vi "Main.vi"() -> ()   [LabVIEW 2015, in "SR430Class.lvclass"]
doc: "This template is for the Queued Message Handler design pattern.\n\nThe Event Handling Loop generates messages based on user interface actions.\n\nThe Message Handling Loop processes messages generated by the Event Handling Loop, or by other messages. The messages are string values, so new messages can be added easily to the Message Cases case structure in the Message Handling Loop. Each message cluster can also provide an optional value for Message Data, which is a variant that can be converted to whatever message-specific data is required."
uses:
  class/SR430Class.lvclass
  support/Type Definitions/Export.ctl
  support/Type Definitions/Mode.ctl
  support/Type Definitions/Schedule.ctl
  support/Type Definitions/saveGraph.ctl
  class/SR430Class.lvclass/SR430Class.ctl
  support/SR430 Driver/SR430_VISA Control.ctl
  support/Message Queue/Enqueue Message (Single).vi
  <vilib>/Utility/error.llb/Error Cluster From Error Code.vi
  <vilib>/ErrorRing/Error Ring.xnode
  support/Message Queue/Message Queue.lvlib
  support/User Event - Stop/User Event - Stop.lvlib
  support/SR430 Driver/SR430Driver.lvlib
  support/Error Handling/Error Handling.lvlib
  support/Type Definitions/Type Definition.lvlib
panel:
  in  "Save":T1
  in  "Schedule":T2 caption="Open"
  in  "Mode":T3 caption="Config"
  in  "Excel Export":T4 caption="New"
  in  "VISA resource name":refnum<visa-resource-name>="Select COM Port"
  in  "Blink":bool caption="Blank"
  in  "Abort":bool
  in  "Accept Mode":bool caption="Blank"
  out "Display":string caption="String"
  in  "Start Timed Acq.":bool caption="Blank"
  in  "TRIGGER LEVEL":dbl=0.1 caption="Numeric" min=-2.0 max=2.0
  in  "DISCRIM. LEVEL":dbl=-0.3 caption="Numeric" min=-0.3 max=0.3
  in  "BINS/RECORD":i32=1 caption="Numeric" min=1 max=16
  in  "RECORDS/SCAN":i32=1000 caption="Numeric" min=0 max=655355
  in  "BIN WIDTH":i32 caption="Numeric" min=0 max=19
  in  "TRIGGER OFFSET":i32=1 caption="Numeric" min=0 max=16384 step=16
  in  "Clock":bool caption="Blank"
  in  "Discrim Slope":bool caption="Blank"
  in  "Trigger Slope":bool=TRUE caption="Blank"
  in  "Startup Banner 2":string="Architect: Ryan J. Richards\nSupervising Professor: Dr. TIm Kane\nThe Pennsylvania State University" caption="String"
  out "ID":string caption="String"
  in  "Startup Banner":string="Stanford Research Systems\nModel SR430 Multi-Channel Scaler | Photon Counter" caption="String"
  in  "Seconds":dbl caption="Numeric" min=0.0
  in  "Minutes":dbl caption="Numeric" min=0.0
  in  "Acquitision Iteration":i32=1 caption="Numeric" min=1
  in  "Hours":dbl caption="Numeric" min=0.0
  out "SR430 Output":dbl[][](graph)
  in  "Clear":bool caption="Reset"
  in  "Pause":bool
  in  "Start":bool
  in  "SR430 Resource":refnum<class "SR430Class.lvclass">
  # "TIMED ACQUISITION"
  # "SYSTEM SETTINGS"
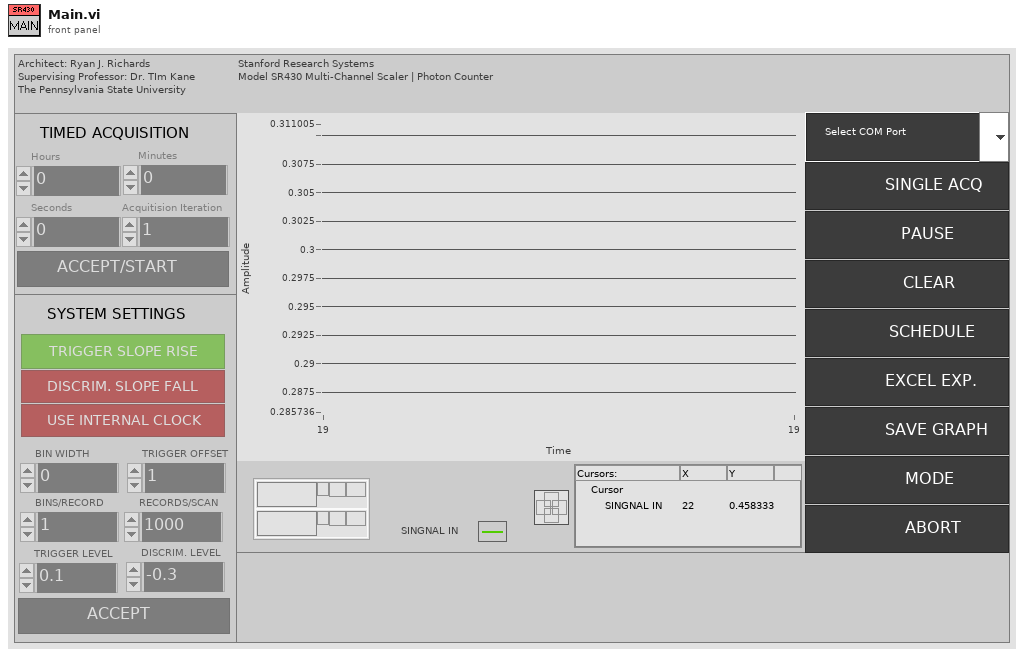
[diagram p1: front panel]
types:
  T1 = typedef "Type Definition.lvlib/saveGraph.ctl" = bool
  T2 = typedef "Type Definition.lvlib/Schedule.ctl" = bool
  T3 = typedef "Type Definition.lvlib/Mode.ctl" = bool
  T4 = typedef "Type Definition.lvlib/Export.ctl" = bool
  T5 = typedef "Message Queue.lvlib/All Message Queues.ctl" = cluster{"UI":refnum<queue>}
  T6 = enum8{"Enabled", "Disabled", "Disabled and Grayed Out"}
  T7 = typedef "SR430Driver.lvlib/SR430_VISA Control.ctl" = cluster{"VISA resource name":refnum<visa-resource-name>}
  T8 = cluster{"Trigger Level (V)":dbl, "Discriminator Level (V)":dbl, "Trigger Slope":bool, "Disc. Slope":bool, "Use External Clock":bool, "Bin Width":i32, "Bins/Record":i32, "Records/Scan":i32, "Trigger Offset":i32}
  T9 = cluster{"Hours":dbl, "Minutes":dbl, "Seconds":dbl, "ACQ #:":i32}
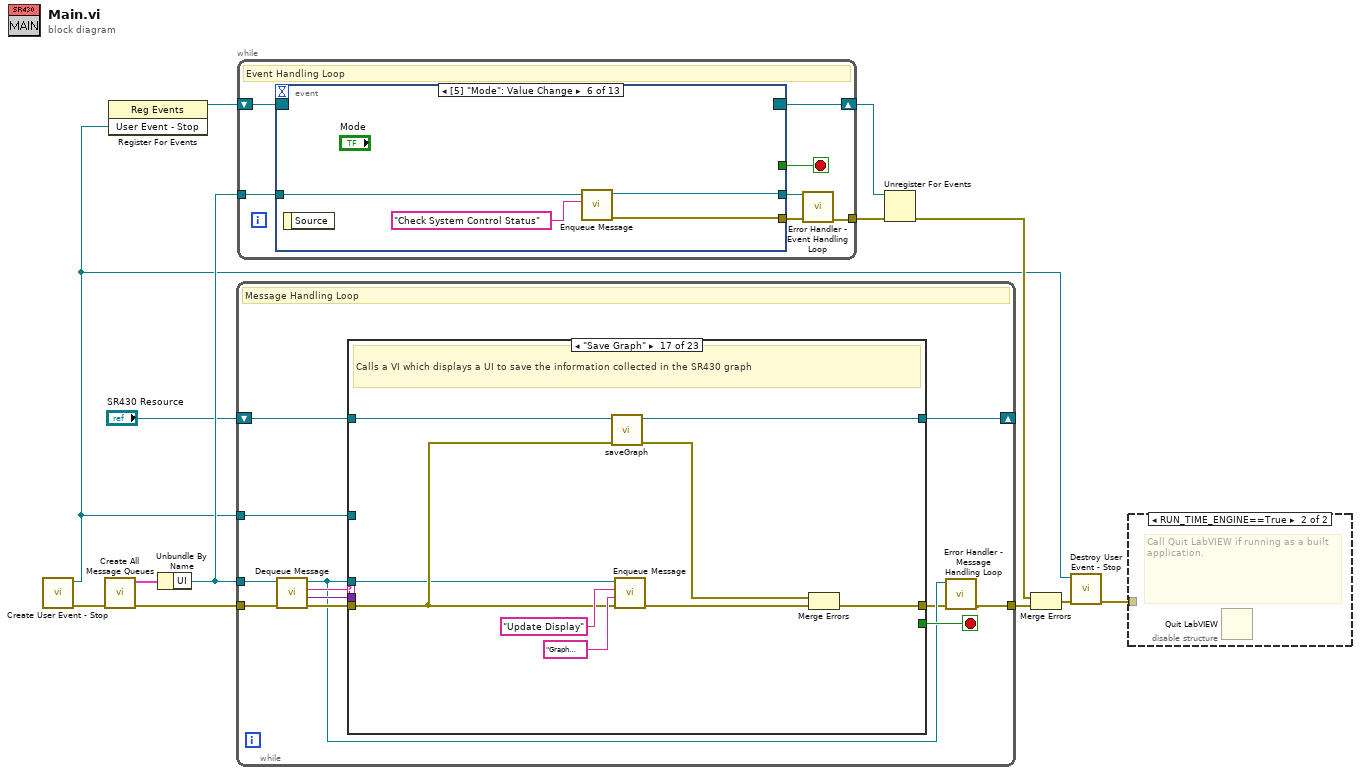
[diagram p0: block diagram]
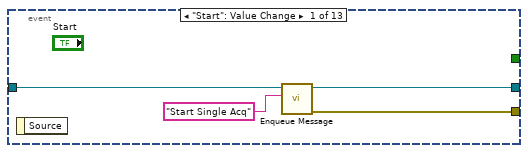
[diagram p3: hidden frame]
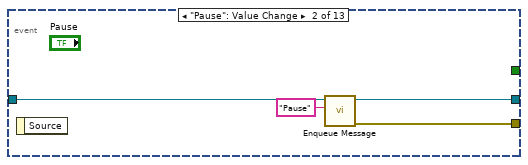
[diagram p4: hidden frame]
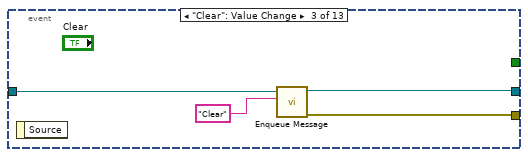
[diagram p5: hidden frame]
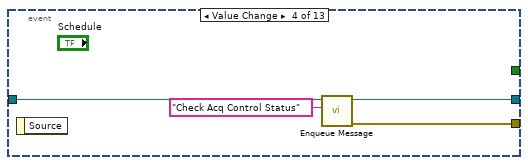
[diagram p6: hidden frame]
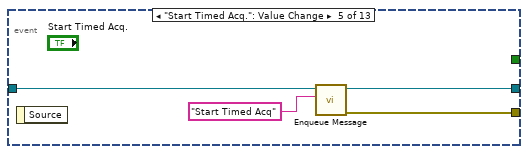
[diagram p7: hidden frame]
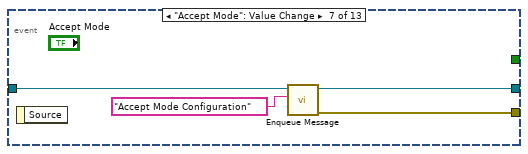
[diagram p8: hidden frame]
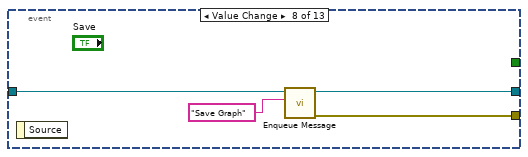
[diagram p9: hidden frame]
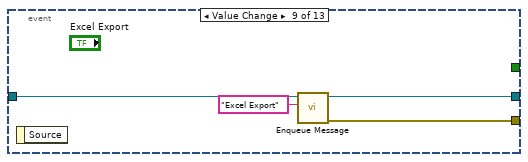
[diagram p10: hidden frame]
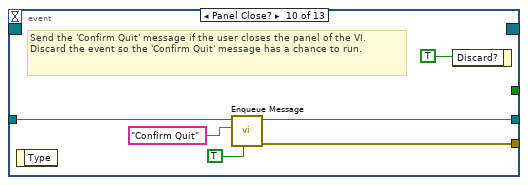
[diagram p11: hidden frame]
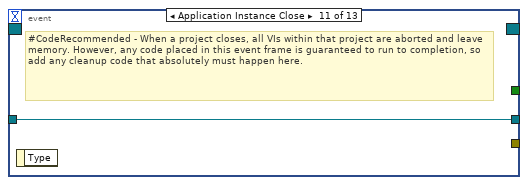
[diagram p12: hidden frame]
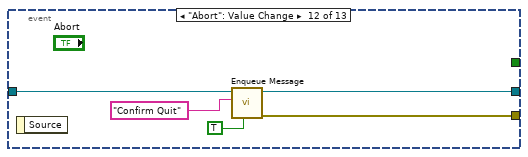
[diagram p13: hidden frame]
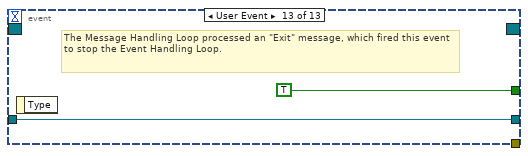
[diagram p14: hidden frame]
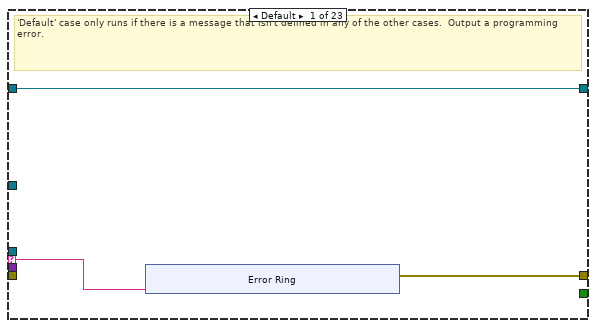
[diagram p15: hidden frame]
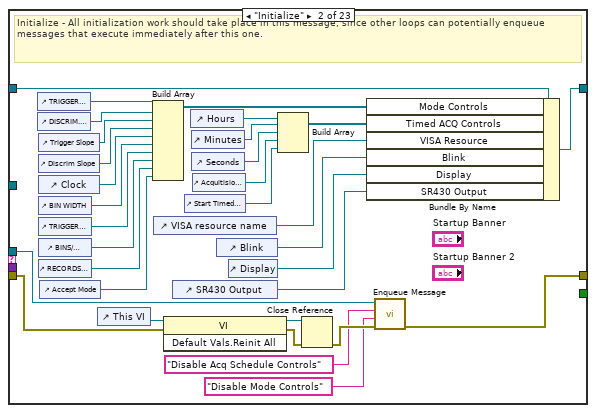
[diagram p16: hidden frame]
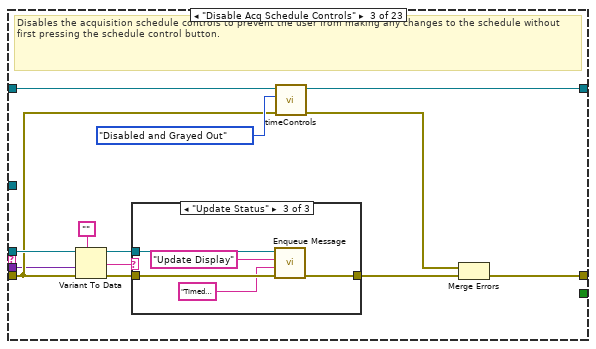
[diagram p17: hidden frame]
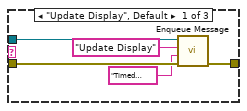
[diagram p18: hidden frame]
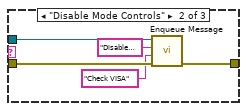
[diagram p19: hidden frame]
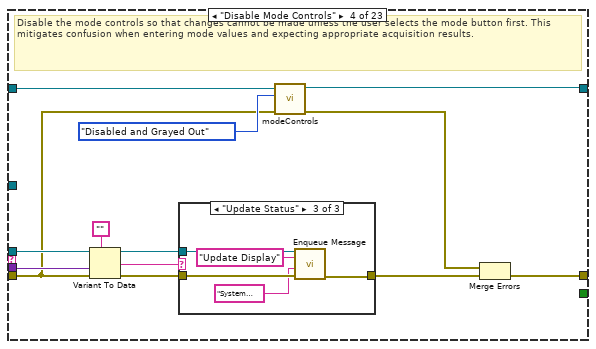
[diagram p20: hidden frame]
diagram:
  n1 = call "Create User Event - Stop.vi"() -> ("error out"=w9:errorcluster, "User Event - Stop"=w3:refnum<user-event>)  [unwired: 10 in]
  n2 = call "Create All Message Queues.vi"("error in (no error)"=w9) -> ("error out"=w13:errorcluster, "Message Queues out"=w12:T5)  [unwired: 9 in]
  n3 = register-events(w3) -> (reference out=w4:refnum<event-registration>)  [unwired: 2 in, 1 out]
  n4 = Unbundle By Name(w12) -> ("UI"=w10:refnum<queue>)
  n5 = while {
    tunnel: w10 -> [w17]
    shift-right: [w24] -> _
    shift-left: "SR430 Resource" -> [w25]
    tunnel: w3 -> [w22]
    tunnel: w13 -> [w21]
    tunnel: [w14] -> w11
    stop <- w23 stop-if-true
    # "Message Handling Loop"
    n6 = call "Dequeue Message.vi"("error in (no error)"=w21, "Message Queue"=w17) -> ("error out"=w20:errorcluster, "Message Data"=w18:variant, "Message"=w19:string, "dup Message Queue"=w16:refnum<queue>)  [unwired: 6 in]
    n7 = case "Message Cases" shown="\"Save Graph\"" w19 {
      selector: w19 -> [w26 _ _ _ _ _ _ _ _ _ _ _ _ _ _ _ _ _ _ _ _ _ _]
      tunnel: w16 -> [_ w59 w70 w103 w126 w144 w155 w170 w178 w188 w215 w226 w234 _ w252 w259 w263 w277 _ w293 _ w306 w328]
      tunnel: w20 -> [_ w64 w69 w96 w125 w143 w150 w166 w177 w187 w216 w222 w235 w245 w251 w260 w266 w278 w285 w292 w303 w305 w321]
      tunnel: [w27 w60 w75 w100 w121 w136 w152 w167 w174 w183 w212 w228 w230 w244 w248 w256 w264 w272 w286 w290 w298 w304 w324] -> w15
      tunnel: w25 -> [w28 w67 w79 w106 w128 w146 w158 w173 w182 w194 w219 w224 w242 w247 w255 w262 w271 w280 w287 w295 w302 w311 w327]
      tunnel: [w28 w66 w78 w105 w127 w145 w157 w172 w181 w193 w218 w223 w241 w246 w254 w262 w270 w279 w287 w294 w302 w311 w327] -> w24
      tunnel: [_ _ _ _ _ _ _ _ _ _ _ _ _ _ _ _ _ _ _ _ _ _ TRUE] -> w23
      tunnel: w18 -> [_ _ w68 w98 _ _ w148 _ _ w186 _ _ _ _ _ _ _ _ w284 _ w301 _ w318]
      tunnel: w22 -> [_ _ _ _ _ _ _ _ _ _ _ _ _ _ _ _ _ _ _ _ _ _ w323]
      frame Default {
        # "'Default' case only runs if there is a message that isn't defined in any of the other cases.  Output a programming error."
        n8 = xnode "Error Ring"("parameter 0"=w26) -> ("error out"=w27:errorcluster)
      }
      frame "Initialize" {
        # "Initialize - All initialization work should take place in this message, since other loops can potentially enqueue messages that execute immediately after this one."
        n9 = control-ref of="TRIGGER LEVEL"() -> (w55:refnum<vi>)
        n10 = control-ref of="DISCRIM. LEVEL"() -> (w54:refnum<vi>)
        n11 = control-ref of="Trigger Slope"() -> (w53:refnum<vi>)
        n12 = control-ref of="Discrim Slope"() -> (w52:refnum<vi>)
        n13 = control-ref of="Clock"() -> (w51:refnum<vi>)
        n14 = control-ref of="BIN WIDTH"() -> (w50:refnum<vi>)
        n15 = control-ref of="TRIGGER OFFSET"() -> (w49:refnum<vi>)
        n16 = control-ref of="BINS/RECORD"() -> (w48:refnum<vi>)
        n17 = control-ref of="RECORDS/SCAN"() -> (w47:refnum<vi>)
        n18 = control-ref of="Accept Mode"() -> (w45:refnum<vi>)
        n19 = control-ref of="This VI"() -> (w65:refnum<vi>)
        n20 = Build Array(w55, w54, w53, w52, w51, w50, w49, w48, w47, w45) -> (w46:refnum<vi>[])
        n21 = control-ref of="VISA resource name"() -> (w57:refnum<vi>)
        n22 = invoke class="VI" method="Default Vals.Reinit All"(reference=w65, error in=w64) -> (reference out=w63:refnum<vi>, error out=w62:errorcluster)  [unwired: 1 in, 1 out]
        n23 = control-ref of="SR430 Output"() -> (w36:refnum<vi>)
        n24 = control-ref of="Start Timed Acq."() -> (w39:refnum<vi>)
        n25 = control-ref of="Hours"() -> (w44:refnum<vi>)
        n26 = control-ref of="Minutes"() -> (w43:refnum<vi>)
        n27 = control-ref of="Seconds"() -> (w42:refnum<vi>)
        n28 = control-ref of="Acquitision Iteration"() -> (w41:refnum<vi>)
        n29 = control-ref of="Blink"() -> (w56:refnum<vi>)
        n30 = control-ref of="Display"() -> (w38:refnum<vi>)
        n31 = Build Array(w44, w43, w42, w41, w39) -> (w40:refnum<vi>[])
        n32 = Close Reference(reference=w63, error in (no error)=w62) -> (error out=w61:errorcluster)
        n33 = Bundle By Name(cluster=w67, "Mode Controls"=w46, "Timed ACQ Controls"=w40, "VISA Resource"=w57, "Blink"=w56, "Display"=w38, "SR430 Output"=w36) -> (w66:refnum<class "SR430Class.lvclass">)
        n34 = call-poly "Enqueue Message.vi"("error in (no error)"=w61, "Message Data"="Disable Mode Controls" ("Message"), "Message"="Disable Acq Schedule Controls", "Message Queue"=w59) -> ("error out"=w60:errorcluster)  [unwired: 6 in, 1 out]
      }
      frame "Disable Acq Schedule Controls" {
        # "Disables the acquisition schedule controls to prevent the user from making any changes to the schedule without first pressing the schedule control button."
        n35 = Variant To Data(error in=w69, type="", Variant=w68) -> (data=w73:string, error out=w72:errorcluster)
        n36 = case shown="\"Update Status\"" w73 {
          tunnel: w72 -> [w83 w89 w94]
          tunnel: w70 -> [w84 w88 w92]
          tunnel: [w81 w86 w93] -> w71
          frame "Update Display", Default {
            n37 = call-poly "Enqueue Message.vi"("error in (no error)"=w83, "Message Data"="Timed acquisition process complete" ("Message"), "Message"="Update Display", "Message Queue"=w84) -> ("error out"=w81:errorcluster)  [unwired: 6 in, 1 out]
          }
          frame "Disable Mode Controls" {
            n38 = call-poly "Enqueue Message.vi"("error in (no error)"=w89, "Message Data"="Check VISA" ("Message"), "Message"="Disable Mode Controls", "Message Queue"=w88) -> ("error out"=w86:errorcluster)  [unwired: 6 in, 1 out]
          }
          frame "Update Status" {
            n39 = call-poly "Enqueue Message.vi"("error in (no error)"=w94, "Message Data"="Timed ACQ Controls Disabled" ("Message"), "Message"="Update Display", "Message Queue"=w92) -> ("error out"=w93:errorcluster)  [unwired: 6 in, 1 out]
          }
        }
        n40 = call-dynamic "timeControls.vi"("error in (no error)"=w69, "Enabled/Disabled"=T6."Disabled and Grayed Out", "SR430Class in"=w79) -> ("error out"=w76:errorcluster, "SR430Class out"=w78:refnum<class "SR430Class.lvclass">)  [unwired: 7 in]
        n41 = Merge Errors(w76, w71) -> (w75:errorcluster)
      }
      frame "Disable Mode Controls" {
        # "Disable the mode controls so that changes cannot be made unless the user selects the mode button first. This mitigates confusion when entering mode values and expecting appropriate acquisition results."
        n42 = Variant To Data(error in=w96, type="", Variant=w98) -> (data=w97:string, error out=w95:errorcluster)
        n43 = case shown="\"Update Status\"" w97 {
          tunnel: w95 -> [w110 w115 w119]
          tunnel: w103 -> [w111 w114 w120]
          tunnel: [w107 w112 w118] -> w102
          frame "Update Display", Default {
            n44 = call-poly "Enqueue Message.vi"("error in (no error)"=w110, "Message Data"="System settings have been updated." ("Message"), "Message"="Update Display", "Message Queue"=w111) -> ("error out"=w107:errorcluster)  [unwired: 6 in, 1 out]
          }
          frame "Check VISA" {
            n45 = call-poly "Enqueue Message.vi"("error in (no error)"=w115, "Message"="Check VISA", "Message Queue"=w114) -> ("error out"=w112:errorcluster)  [unwired: 7 in, 1 out]
          }
          frame "Update Status" {
            n46 = call-poly "Enqueue Message.vi"("error in (no error)"=w119, "Message Data"="System settings controls disabled." ("Message"), "Message"="Update Display", "Message Queue"=w120) -> ("error out"=w118:errorcluster)  [unwired: 6 in, 1 out]
          }
        }
        n47 = call "modeControls.vi"("error in (no error)"=w96, "Enabled/Disabled"=T6."Disabled and Grayed Out", "SR430Class in"=w106) -> ("error out"=w101:errorcluster, "SR430Class out"=w105:refnum<class "SR430Class.lvclass">)  [unwired: 7 in]
        n48 = Merge Errors(w101, w102) -> (w100:errorcluster)
      }
      frame "Check VISA" {
        # "Checks the VISA control to determine whether or not a COM port has been selected (other than default value). If it has not then the control will blink and require the user to change the port and select a valid one"
        n49 = call-dynamic "checkVisa.vi"("error in (no error)"=w125, "SR430Class in"=w128) -> ("error out"=w123:errorcluster, "SR430Class out"=w127:refnum<class "SR430Class.lvclass">)  [unwired: 8 in]
        n50 = call-poly "Enqueue Message.vi"("error in (no error)"=w125, "Message"="Initialize SR430", "Message Queue"=w126) -> ("error out"=w122:errorcluster)  [unwired: 7 in, 1 out]
        n51 = Merge Errors(w123, w122) -> (w121:errorcluster)
      }
      frame "Initialize SR430" {
        # "Provide the VISA resource so that the SR430 can connect to LabVIEW. The connection status and identification number is then displayed accordingly."
        n52 = Bundle By Name(cluster=T7 {"VISA resource name"=""} ("SR430 VISA Cluster"), "VISA resource name"="VISA resource name") -> (w129:T7)
        n53 = call-dynamic "initializeSR430.vi"("error in (no error)"=w143, "SR430 VISA Cluster"=w129, "dataClass in"=w146) -> ("error out"=w135:errorcluster, "ID #:"=w133:string, "Connected"=w141:bool, "dataClass out"=w145:refnum<class "SR430Class.lvclass">)  [unwired: 5 in]
        n54 = Select(t="Connected to SR430" ("Message"), s=w141, f="Failed to connect to SR430" ("Message")) -> (s? t:f=w139:string)
        n55 = Concatenate Strings("Connected to:" ("string"), w133) -> (→"ID":string)
        n56 = call-poly "Enqueue Message.vi"("error in (no error)"=w143, "Message Data"=w139, "Message"="Update Display", "Message Queue"=w144) -> ("error out"=w137:errorcluster)  [unwired: 6 in, 1 out]
        n57 = Merge Errors(w135, w137) -> (w136:errorcluster)
      }
      frame "Enable Mode Controls" {
        # "Enable Mode Controls so that the user can change them and ultimately accept the configuration. This prevents the user from changing them during execution and mitigates confusion and error."
        n58 = Variant To Data(error in=w150, type="", Variant=w148) -> (data=w147:string, error out=w149:errorcluster)
        n59 = case shown="\"Update Status\"" w147 {
          tunnel: w149 -> [w159 w164]
          tunnel: w155 -> [_ w163]
          tunnel: [w159 w160] -> w154
          frame Default {
          }
          frame "Update Status" {
            n60 = call-poly "Enqueue Message.vi"("error in (no error)"=w164, "Message Data"="System settings controls enabled." ("Message"), "Message"="Update Display", "Message Queue"=w163) -> ("error out"=w160:errorcluster)  [unwired: 6 in, 1 out]
          }
        }
        n61 = call "modeControls.vi"("error in (no error)"=w150, "Enabled/Disabled"=T6."Enabled", "SR430Class in"=w158) -> ("error out"=w153:errorcluster, "SR430Class out"=w157:refnum<class "SR430Class.lvclass">)  [unwired: 7 in]
        n62 = Merge Errors(w153, w154) -> (w152:errorcluster)
      }
      frame "Check Acq Control Status" {
        # "Checks the status of the acquisition controls and reads whether they are enabled or disabled - then assigns the next state accordingly."
        n63 = call-dynamic "CheckControlStatus.vi"("error in (no error)"=w166, "SR430Class in"=w173) -> ("error out"=w168:errorcluster, "Enable/Disable Controls"=w171:string, "SR430Class out"=w172:refnum<class "SR430Class.lvclass">)  [unwired: 7 in]
        n64 = call-poly "Enqueue Message.vi"("error in (no error)"=w166, "Message Data"="Update Status" ("Enable/Disable Controls"), "Message"=w171, "Message Queue"=w170) -> ("error out"=w169:errorcluster)  [unwired: 6 in, 1 out]
        n65 = Merge Errors(w168, w169) -> (w167:errorcluster)
      }
      frame "Check System Control Status" {
        # "Checks the status of the system settings controls and reads whether they are enabled or disabled - then assigns the next state accordingly."
        n66 = call-dynamic "CheckSystemSettingControl.vi"("error in (no error)"=w177, "SR430Class in"=w182) -> ("error out"=w176:errorcluster, "Enable/Disable Controls"=w179:string, "SR430Class out"=w181:refnum<class "SR430Class.lvclass">)  [unwired: 7 in]
        n67 = call-poly "Enqueue Message.vi"("error in (no error)"=w177, "Message Data"="Update Status" ("Enable/Disable Controls"), "Message"=w179, "Message Queue"=w178) -> ("error out"=w175:errorcluster)  [unwired: 6 in, 1 out]
        n68 = Merge Errors(w176, w175) -> (w174:errorcluster)
      }
      frame "Enable Acq Schedule Controls" {
        # "Enables the acqusition schedule controls so that the user can enter the desired time values and execute the acquisition process."
        n69 = Variant To Data(error in=w187, type="", Variant=w186) -> (data=w190:string, error out=w189:errorcluster)
        n70 = case shown="\"Update Status\"" w190 {
          tunnel: w189 -> [w195 w200]
          tunnel: w188 -> [_ w198]
          tunnel: [w195 w199] -> w185
          frame Default {
          }
          frame "Update Status" {
            n71 = call-poly "Enqueue Message.vi"("error in (no error)"=w200, "Message Data"="Timed ACQ Controls Enabled." ("Message"), "Message"="Update Display", "Message Queue"=w198) -> ("error out"=w199:errorcluster)  [unwired: 6 in, 1 out]
          }
        }
        n72 = call-dynamic "timeControls.vi"("error in (no error)"=w187, "Enabled/Disabled"=T6."Enabled", "SR430Class in"=w194) -> ("error out"=w184:errorcluster, "SR430Class out"=w193:refnum<class "SR430Class.lvclass">)  [unwired: 7 in]
        n73 = Merge Errors(w184, w185) -> (w183:errorcluster)
      }
      frame "Accept Mode Configuration" {
        # "Writes the mode values to the SR430, effectively updating the settings on the device so that a specific acquisition can be completed."
        n74 = Bundle By Name(cluster=T8 {"Trigger Level (V)"=0.1, "Discriminator Level (V)"=-0.3, "Trigger Slope"=FALSE, "Disc. Slope"=TRUE, "Use External Clock"=FALSE, "Bin Width"=0, "Bins/Record"=1, "Records/Scan"=1000, "Trigger Offset"=0}, "Trigger Level (V)"="TRIGGER LEVEL", "Discriminator Level (V)"="DISCRIM. LEVEL", "Trigger Slope"="Trigger Slope", "Disc. Slope"="Discrim Slope", "Use External Clock"="Clock", "Bin Width"="BIN WIDTH", "Bins/Record"="BINS/RECORD", "Records/Scan"="RECORDS/SCAN", "Trigger Offset"="TRIGGER OFFSET") -> (w217:T8)
        n75 = call-dynamic "acceptMode.vi"("error in (no error)"=w216, "Mode Controls"=w217, "SR430Class in"=w219) -> ("error out"=w213:errorcluster, "SR430Class out"=w218:refnum<class "SR430Class.lvclass">)  [unwired: 7 in]
        n76 = call-poly "Enqueue Message.vi"("error in (no error)"=w216, "Message Data"="Update Display" ("Message"), "Message"="Disable Mode Controls", "Message Queue"=w215) -> ("error out"=w214:errorcluster)  [unwired: 6 in, 1 out]
        n77 = Merge Errors(w213, w214) -> (w212:errorcluster)
      }
      frame "Start Single Acq" {
        # "Start single data acquisition then shows the results on the waveform graph (processed in the \"Show Output\" case)"
        n78 = call-dynamic "Play.vi"("error in (no error)"=w222, "Data in"=w224) -> ("error out"=w221:errorcluster, "Data out"=w223:refnum<class "SR430Class.lvclass">)  [unwired: 8 in]
        n79 = call-poly "Enqueue Message.vi"("error in (no error)"=w222, "Message"="Show Output", "Message Queue"=w226) -> ("error out"=w227:errorcluster)  [unwired: 7 in, 1 out]
        n80 = Merge Errors(w221, w227) -> (w228:errorcluster)
      }
      frame "Start Timed Acq" {
        # "Starts the timed acquisition process based on the user's time parameters. The time indicators are updated constantly so that the user is informed of the duration of the acquisition process."
        n81 = Bundle By Name(cluster=T9 {"Hours"=0.0, "Minutes"=0.0, "Seconds"=0.0, "ACQ #:"=0}, "Hours"="Hours", "Minutes"="Minutes", "Seconds"="Seconds", "ACQ #:"="Acquitision Iteration") -> (w240:T9)
        n82 = call-dynamic "timedAcq.vi"("error in (no error)"=w235, "Time Controls"=w240, "SR430Class in"=w242) -> ("error out"=w232:errorcluster, "SR430Class out"=w241:refnum<class "SR430Class.lvclass">)  [unwired: 7 in]
        n83 = call-poly "Enqueue Message.vi"("error in (no error)"=w235, "Message Data"="Update Display" ("Message"), "Message"="Disable Acq Schedule Controls", "Message Queue"=w234) -> ("error out"=w231:errorcluster)  [unwired: 6 in, 1 out]
        n84 = Merge Errors(w232, w231) -> (w230:errorcluster)
      }
      frame "Pause" {
        # "Pauses the data acquistion process to prevent more data from being collected."
        n85 = call-dynamic "Pause.vi"("error in (no error)"=w245, "SR430Class in"=w247) -> ("error out"=w244:errorcluster, "SR430Class out"=w246:refnum<class "SR430Class.lvclass">)  [unwired: 8 in]
      }
      frame "Clear" {
        # "Clears the SR430 display so that new information can be collected and displayed. This does not need to be pressed before the data acquisition. The clear function is built into the acquisition process."
        n86 = call-dynamic "Clear.vi"("error in (no error)"=w251, "dataClass in"=w255) -> ("error out"=w249:errorcluster, "dataClass out"=w254:refnum<class "SR430Class.lvclass">)  [unwired: 8 in]
        n87 = call-poly "Enqueue Message.vi"("error in (no error)"=w251, "Message"="Show Output", "Message Queue"=w252) -> ("error out"=w250:errorcluster)  [unwired: 7 in, 1 out]
        n88 = Merge Errors(w249, w250) -> (w248:errorcluster)
      }
      frame "Show Output" {
        # "Show the data that the SR430 has collected."
        n89 = Unbundle By Name(w262) -> ("SR430 Data"=→"SR430 Output":dbl[][])
        n90 = call-poly "Enqueue Message.vi"("error in (no error)"=w260, "Message Data"="SR430 graph updated." ("Message"), "Message"="Update Display", "Message Queue"=w259) -> ("error out"=w256:errorcluster)  [unwired: 6 in, 1 out]
      }
      frame "Save Graph" {
        # "Calls a VI which displays a UI to save the information collected in the SR430 graph"
        n91 = call-dynamic "saveGraph.vi"("error in (no error)"=w266, "SR430 Resource in"=w271) -> ("error out"=w265:errorcluster, "SR430 Resource out"=w270:refnum<class "SR430Class.lvclass">)  [unwired: 8 in]
        n92 = call-poly "Enqueue Message.vi"("error in (no error)"=w266, "Message Data"="Graph successfully saved." ("Message"), "Message"="Update Display", "Message Queue"=w263) -> ("error out"=w267:errorcluster)  [unwired: 6 in, 1 out]
        n93 = Merge Errors(w265, w267) -> (w264:errorcluster)
      }
      frame "Excel Export" {
        # "Exports all collected data to a user-defined Excel spreadsheet."
        n94 = call "excelExport.vi"("error in (no error)"=w278, "SR430Class.lvclass (in)"=w280) -> ("error out"=w273:errorcluster, "SR430Class.lvclass (out)"=w279:refnum<class "SR430Class.lvclass">)  [unwired: 8 in]
        n95 = call-poly "Enqueue Message.vi"("error in (no error)"=w278, "Message Data"="Excel file successfully created." ("Message"), "Message"="Update Display", "Message Queue"=w277) -> ("error out"=w274:errorcluster)  [unwired: 6 in, 1 out]
        n96 = Merge Errors(w273, w274) -> (w272:errorcluster)
      }
      frame "Update Display" {
        # "Update Display - Convert the message data to a string to display in the Data Display indicator."
        n97 = Variant To Data(error in=w285, type="", Variant=w284) -> (data=→"Display":string, error out=w282:errorcluster)
        n98 = Merge Errors(w282) -> (w286:errorcluster)
      }
      frame "Close Resource" {
        # "Closes the SR430 VISA resource to ensure that the connection is properly terminated, allowing future sessions to mitigate VISA resource error."
        n99 = call-dynamic "closeResource.vi"("error in (no error)"=w292, "SR430Class in"=w295) -> ("error out"=w289:errorcluster, "SR430Class out"=w294:refnum<class "SR430Class.lvclass">)  [unwired: 8 in]
        n100 = call-poly "Enqueue Message.vi"("error in (no error)"=w292, "Message"="Exit", "Message Queue"=w293) -> ("error out"=w291:errorcluster)  [unwired: 7 in, 1 out]
        n101 = Merge Errors(w289, w291) -> (w290:errorcluster)
      }
      frame "Error" {
        # "Error - Display an error dialog. This message is sent by the \"Error Handler\" VIs at the end of other loops in this application."
        n102 = Variant To Data(error in=w303, type=errorcluster {"status"=FALSE, "code"=0, "source"=""} ("error constant"), Variant=w301) -> (data=w297:errorcluster, error out=w299:errorcluster)
        n103 = call "SR430 Error Message.vi"("error in (no error)"=w297) -> ("error out"=w296:errorcluster)  [unwired: 15 in, 3 out]
        n104 = Merge Errors(w296, w299) -> (w298:errorcluster)
      }
      frame "Confirm Quit" {
        # "Confirm Quit - Message that can confirm whether or not the user wants to exit the application."
        n105 = Two Button Dialog(message="Are you sure that you want to abort the sequence?", 1:"NO" ("F button name (\"Cancel\")"), 2:"YES" ("T button name (\"OK\")")) -> (T button?=w310:bool)
        n106 = case shown="True" w310 {
          tunnel: w305 -> [w312 w317]
          tunnel: [w312 w313] -> w304
          tunnel: w306 -> [_ w316]
          frame False {
          }
          frame True {
            n107 = call-poly "Enqueue Message.vi"("Priority Message? (F)"=TRUE, "error in (no error)"=w317, "Message"="Close Resource", "Message Queue"=w316) -> ("error out"=w313:errorcluster)  [unwired: 6 in, 1 out]
          }
        }
      }
      frame "Exit" {
        # "Exit - Exit the application."
        n108 = Variant To Data(type=errorcluster {"status"=FALSE, "code"=0, "source"=""} ("error constant"), Variant=w318) -> (data=w319:errorcluster)  [unwired: 1 in, 1 out]
        n109 = call <vilib>:"Simple Error Handler.vi"("error in (no error)"=w319) -> ()  [unwired: 4 in, 5 out]
        n110 = call "Fire User Event - Stop.vi"("User Event - Stop"=w323) -> ("error out"=w322:errorcluster)  [unwired: 10 in]
        n111 = Release Queue(queue=w328, error in (no error)=w321) -> (error out=w325:errorcluster)  [unwired: 1 in, 2 out]
        n112 = Merge Errors(w322, w325) -> (w324:errorcluster)
      }
    }
    n113 = call "Error Handler - Message Handling Loop.vi"("error in (no error)"=w15, "Message Queue"=w16) -> ("dup error in"=w14:errorcluster)  [unwired: 8 in, 1 out]
  }
  n114 = while {
    tunnel: w10 -> [w335]
    shift-right: [w333] -> w6
    shift-left: w4 -> [w334]
    tunnel: [w329] -> w5
    stop <- w332 stop-if-true
    # "Event Handling Loop"
    n115 = event shown="[5] \"Mode\": Value Change" {
      selector: w334 -> [_ _ _ _ _ _ _ _ _ _ _ _ _]
      dyn-events: [_ _ _ _ _ _ _ _ _ _ _ _ _] -> w333
      timeout: _ -> [_ _ _ _ _ _ _ _ _ _ _ _ _]
      tunnel: [_ _ _ _ _ _ _ _ _ _ _ _ TRUE ("Discard?")] -> w332
      tunnel: w335 -> [w339 w343 w347 w351 w355 w359 w363 w367 w371 w376 w378 w383 w385]
      tunnel: [w336 w341 w345 w348 w353 w357 w361 w365 w369 w375 _ w382 _] -> w330
      tunnel: [w338 w342 w346 w350 w354 w358 w362 w366 w370 w374 w378 w381 w385] -> w331
      event "Start": Value Change {
        n116 = event-data() -> ()  [unwired: 1 in, 1 out]
        n117 = call-poly "Enqueue Message.vi"("Message"="Start Single Acq", "Message Queue"=w339) -> ("error out"=w336:errorcluster, "dup Message Queue"=w338:refnum<queue>)  [unwired: 8 in]
      }
      event "Pause": Value Change {
        n118 = event-data() -> ()  [unwired: 1 in, 1 out]
        n119 = call-poly "Enqueue Message.vi"("Message"="Pause", "Message Queue"=w343) -> ("error out"=w341:errorcluster, "dup Message Queue"=w342:refnum<queue>)  [unwired: 8 in]
      }
      event "Clear": Value Change {
        n120 = event-data() -> ()  [unwired: 1 in, 1 out]
        n121 = call-poly "Enqueue Message.vi"("Message"="Clear", "Message Queue"=w347) -> ("error out"=w345:errorcluster, "dup Message Queue"=w346:refnum<queue>)  [unwired: 8 in]
      }
      event Value Change {
        n122 = event-data() -> ()  [unwired: 1 in, 1 out]
        n123 = call-poly "Enqueue Message.vi"("Message"="Check Acq Control Status", "Message Queue"=w351) -> ("error out"=w348:errorcluster, "dup Message Queue"=w350:refnum<queue>)  [unwired: 8 in]
      }
      event "Start Timed Acq.": Value Change {
        n124 = event-data() -> ()  [unwired: 1 in, 1 out]
        n125 = call-poly "Enqueue Message.vi"("Message"="Start Timed Acq", "Message Queue"=w355) -> ("error out"=w353:errorcluster, "dup Message Queue"=w354:refnum<queue>)  [unwired: 8 in]
      }
      event Value Change {
        n126 = event-data() -> ()  [unwired: 1 in, 1 out]
        n127 = call-poly "Enqueue Message.vi"("Message"="Check System Control Status", "Message Queue"=w359) -> ("error out"=w357:errorcluster, "dup Message Queue"=w358:refnum<queue>)  [unwired: 8 in]
      }
      event "Accept Mode": Value Change {
        n128 = event-data() -> ()  [unwired: 1 in, 1 out]
        n129 = call-poly "Enqueue Message.vi"("Message"="Accept Mode Configuration", "Message Queue"=w363) -> ("error out"=w361:errorcluster, "dup Message Queue"=w362:refnum<queue>)  [unwired: 8 in]
      }
      event Value Change {
        n130 = event-data() -> ()  [unwired: 1 in, 1 out]
        n131 = call-poly "Enqueue Message.vi"("Message"="Save Graph", "Message Queue"=w367) -> ("error out"=w365:errorcluster, "dup Message Queue"=w366:refnum<queue>)  [unwired: 8 in]
      }
      event Value Change {
        n132 = event-data() -> ()  [unwired: 1 in, 1 out]
        n133 = call-poly "Enqueue Message.vi"("Message"="Excel Export", "Message Queue"=w371) -> ("error out"=w369:errorcluster, "dup Message Queue"=w370:refnum<queue>)  [unwired: 8 in]
      }
      event Panel Close? {
        # "Send the 'Confirm Quit' message if the user closes the panel of the VI. Discard the event so the 'Confirm Quit' message has a chance to run."
        n134 = event-data() -> ()  [unwired: 1 in, 1 out]
        n135 = call-poly "Enqueue Message.vi"("Priority Message? (F)"=TRUE, "Message"="Confirm Quit", "Message Queue"=w376) -> ("error out"=w375:errorcluster, "dup Message Queue"=w374:refnum<queue>)  [unwired: 7 in]
        n136 = event-data("Discard?"=TRUE) -> ()  [unwired: 1 in, 1 out]
      }
      event Application Instance Close {
        # "#CodeRecommended - When a project closes, all VIs within that project are aborted and leave memory. However, any code placed in this event frame is guaranteed to run to completion, so add any cleanup code that absolutely must happen here."
        n137 = event-data() -> ()  [unwired: 1 in, 1 out]
      }
      event "Abort": Value Change {
        n138 = event-data() -> ()  [unwired: 1 in, 1 out]
        n139 = call-poly "Enqueue Message.vi"("Priority Message? (F)"=TRUE, "Message"="Confirm Quit", "Message Queue"=w383) -> ("error out"=w382:errorcluster, "dup Message Queue"=w381:refnum<queue>)  [unwired: 7 in]
      }
      event User Event {
        # "The Message Handling Loop processed an \"Exit\" message, which fired this event to stop the Event Handling Loop."
        n140 = event-data() -> ()  [unwired: 1 in, 1 out]
      }
    }
    n141 = call "Error Handler - Event Handling Loop.vi"("error in (no error)"=w330, "Message Queue"=w331) -> ("dup error in"=w329:errorcluster)  [unwired: 8 in, 1 out]
  }
  n142 = Unregister For Events(event registration refnum=w6, error in=w5) -> (error out=w7:errorcluster)
  n143 = Merge Errors(w7, w11) -> (w8:errorcluster)
  n144 = call "Destroy User Event - Stop.vi"("error in (no error)"=w8, "User Event - Stop"=w3) -> ("error out"=w2:errorcluster)  [unwired: 9 in]
  n145 = disable-structure shown="RUN_TIME_ENGINE==True" {
    disable-tunnel: w2 -> [_ _]
    frame condition #0 (active) {
    }
    frame condition #1 {
      # "Call Quit LabVIEW if running as a built application."
      n146 = Quit LabVIEW() -> ()  [unwired: 1 in]
    }
  }
